vi "A33Initialize.vi"(8 "error in (no error)":errorcluster, 9 "Reset (True)":bool=TRUE, 11 "VISA resource name":refnum<visa-resource-name>) -> (0 "error out":errorcluster, 3 "VISA resource name out":refnum<visa-resource-name>)   [LabVIEW 2022 SP3]
doc: "Establishes communication with the instrument and optionally performs an instrument identification query and/or an instrument reset. It also places the instrument in a default state needed for other instrument driver operations. Therefore, call this VI before calling other instrument driver VIs for this instrument. Generally, you need to call the Initialize VI only once at the beginning of an application."
panel:
  # "(c) 2008 National Instruments.  ALL RIGHTS RESERVED."
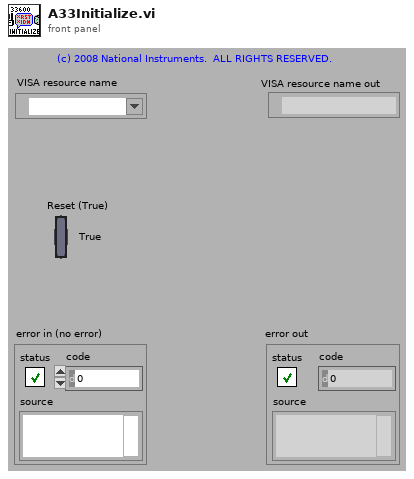
[diagram p1: front panel]
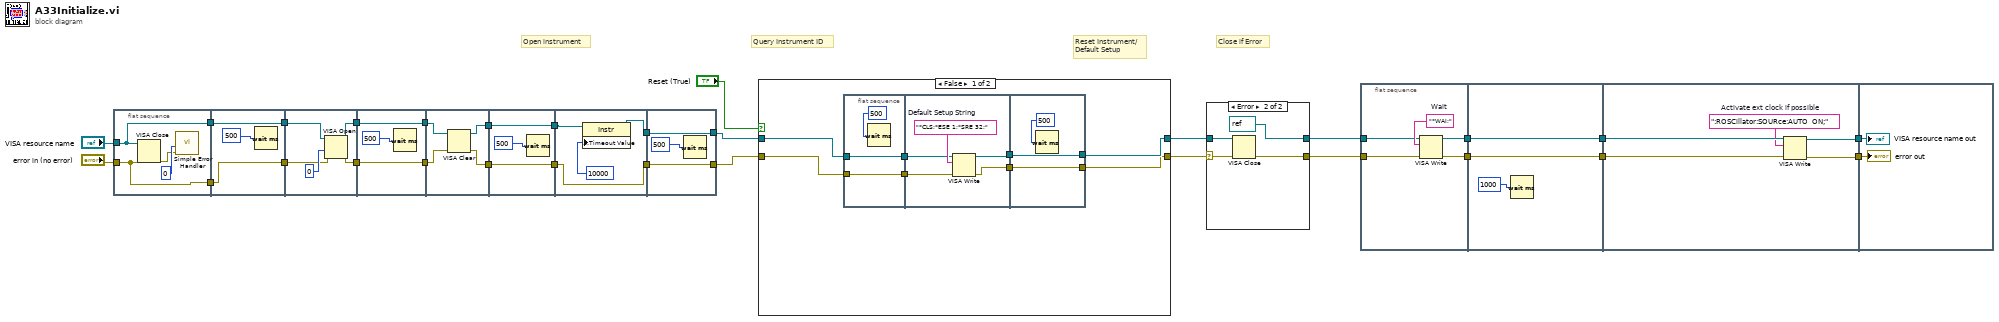
[diagram p0: block diagram]
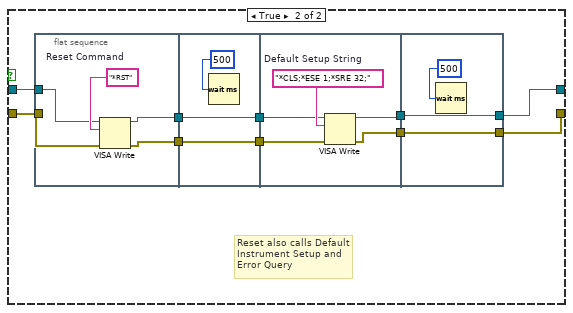
[diagram p3: hidden frame]
diagram:
  # "Close if Error"
  # "Query Instrument ID"
  # "Reset Instrument/\nDefault Setup"
  # "Open instrument"
  n1 = flat-sequence {
    tunnel: "error in (no error)" -> [w31]
    tunnel: "VISA resource name" -> [w30]
    tunnel: [w31] -> w22
    tunnel: [w30] -> w21
    tunnel: w22 -> [w35]
    tunnel: w21 -> [w34]
    tunnel: [w35] -> w20
    tunnel: [w34] -> w19
    tunnel: w20 -> [w39]
    tunnel: w19 -> [w40]
    tunnel: [w38] -> w18
    tunnel: [w37] -> w17
    tunnel: w18 -> [w44]
    tunnel: w17 -> [w43]
    tunnel: [w44] -> w16
    tunnel: [w43] -> w15
    tunnel: w16 -> [w47]
    tunnel: w15 -> [w48]
    tunnel: [w46] -> w14
    tunnel: [w45] -> w13
    tunnel: w14 -> [w51]
    tunnel: w13 -> [w50]
    tunnel: [w51] -> w12
    tunnel: [w50] -> w11
    tunnel: w12 -> [w54]
    tunnel: w11 -> [w53]
    tunnel: [w53] -> w10
    tunnel: [w52] -> w9
    tunnel: [w57] -> w8
    tunnel: [w58] -> w7
    tunnel: w10 -> [w58]
    tunnel: w9 -> [w57]
    frame #0 {
      n2 = VISA Close(VISA resource name=w30, error in (no error)=w31) -> (error out=w32:errorcluster)
      n3 = call <vilib>:"Simple Error Handler.vi"("type of dialog (OK msg:1)"=0, "error in (no error)"=w32) -> ()  [unwired: 3 in, 5 out]
    }
    frame #1 {
      n4 = Wait (ms)(milliseconds to wait=500) -> ()  [unwired: 1 out]
    }
    frame #2 {
      n5 = VISA Open(access mode=u32 0, error in (no error)=w39, VISA resource name=w40) -> (VISA resource name=w37:refnum<visa-resource-name>, error out=w38:errorcluster)  [unwired: 2 in]
    }
    frame #3 {
      n6 = Wait (ms)(milliseconds to wait=500) -> ()  [unwired: 1 out]
    }
    frame #4 {
      n7 = VISA Clear(VISA resource name=w48, error in (no error)=w47) -> (VISA resource name out=w46:refnum<visa-resource-name>, error out=w45:errorcluster)
    }
    frame #5 {
      n8 = Wait (ms)(milliseconds to wait=500) -> ()  [unwired: 1 out]
    }
    frame #6 {
      n9 = property class="Instr"(reference=w54, "General Settings:Timeout Value"=u32 10000) -> (reference out=w52:refnum<visa-resource-name>)  [unwired: 1 in, 1 out]
    }
    frame #7 {
      n10 = Wait (ms)(milliseconds to wait=500) -> ()  [unwired: 1 out]
    }
  }
  n11 = case shown="False" "Reset (True)" {
    tunnel: w7 -> [w61 w86]
    tunnel: [w59 w84] -> w27
    tunnel: w8 -> [w62 w87]
    tunnel: [w60 w85] -> w28
    frame False {
      n12 = flat-sequence {
        tunnel: [w67] -> w66
        tunnel: [w68] -> w65
        tunnel: w62 -> [w67]
        tunnel: w61 -> [w68]
        tunnel: w66 -> [w71]
        tunnel: w65 -> [w70]
        tunnel: [w73] -> w64
        tunnel: [w72] -> w63
        tunnel: [w76] -> w59
        tunnel: [w77] -> w60
        tunnel: w64 -> [w77]
        tunnel: w63 -> [w76]
        frame #0 {
          n13 = Wait (ms)(milliseconds to wait=500) -> ()  [unwired: 1 out]
        }
        frame #1 {
          w74 = "*CLS;*ESE 1;*SRE 32;"  # Default Setup String
          n14 = VISA Write(VISA resource name=w71, write buffer=w74, error in (no error)=w70) -> (VISA resource name out=w73:refnum<visa-resource-name>, error out=w72:errorcluster)  [unwired: 1 out]
        }
        frame #2 {
          n15 = Wait (ms)(milliseconds to wait=500) -> ()  [unwired: 1 out]
        }
      }
    }
    frame True {
      # "Reset also calls Default Instrument Setup and Error Query"
      n16 = flat-sequence {
        tunnel: w87 -> [w91]
        tunnel: w86 -> [w90]
        tunnel: [w89] -> w82
        tunnel: [w88] -> w80
        tunnel: [w95] -> w83
        tunnel: w82 -> [w95]
        tunnel: [w94] -> w81
        tunnel: w80 -> [w94]
        tunnel: w83 -> [w97]
        tunnel: w81 -> [w96]
        tunnel: [w99] -> w79
        tunnel: [w98] -> w78
        tunnel: [w102] -> w84
        tunnel: [w103] -> w85
        tunnel: w79 -> [w103]
        tunnel: w78 -> [w102]
        frame #0 {
          w92 = "*RST"  # Reset Command
          n17 = VISA Write(VISA resource name=w91, write buffer=w92, error in (no error)=w90) -> (VISA resource name out=w89:refnum<visa-resource-name>, error out=w88:errorcluster)  [unwired: 1 out]
        }
        frame #1 {
          n18 = Wait (ms)(milliseconds to wait=500) -> ()  [unwired: 1 out]
        }
        frame #2 {
          w100 = "*CLS;*ESE 1;*SRE 32;"  # Default Setup String
          n19 = VISA Write(VISA resource name=w97, write buffer=w100, error in (no error)=w96) -> (VISA resource name out=w99:refnum<visa-resource-name>, error out=w98:errorcluster)  [unwired: 1 out]
        }
        frame #3 {
          n20 = Wait (ms)(milliseconds to wait=500) -> ()  [unwired: 1 out]
        }
      }
    }
  }
  n21 = case shown="Error" w27 {
    selector: w27 -> [w104 w107]
    tunnel: w28 -> [w105 w108]
    tunnel: [w105 refnum<visa-resource-name> refnum ("VISA resource name out")] -> w26
    tunnel: [w104 w106] -> w25
    frame No Error {
    }
    frame Error {
      n22 = VISA Close(VISA resource name=w108, error in (no error)=w107) -> (error out=w106:errorcluster)
    }
  }
  n23 = flat-sequence {
    tunnel: w25 -> [w112]
    tunnel: w26 -> [w113]
    tunnel: [w111] -> w6
    tunnel: [w110] -> w5
    tunnel: w6 -> [w117]
    tunnel: w5 -> [w116]
    tunnel: [w117] -> w4
    tunnel: [w116] -> w2
    tunnel: w4 -> [w122]
    tunnel: [w120] -> w3
    tunnel: w2 -> [w121]
    tunnel: [w119] -> w1
    tunnel: w3 -> [w124]
    tunnel: w1 -> [w123]
    frame #0 {
      w114 = "*WAI;"  # Wait
      n24 = VISA Write(VISA resource name=w113, write buffer=w114, error in (no error)=w112) -> (VISA resource name out=w111:refnum<visa-resource-name>, error out=w110:errorcluster)  [unwired: 1 out]
    }
    frame #1 {
      n25 = Wait (ms)(milliseconds to wait=1000) -> ()  [unwired: 1 out]
    }
    frame #2 {
      w118 = ":ROSCillator:SOURce:AUTO  ON;"  # Activate ext clock if possible
      n26 = VISA Write(VISA resource name=w122, write buffer=w118, error in (no error)=w121) -> (VISA resource name out=w120:refnum<visa-resource-name>, error out=w119:errorcluster)  [unwired: 1 out]
    }
    frame #3 {
      "VISA resource name out" <- w124
      "error out" <- w123
    }
  }
